vi "Temperature Control.vi"() -> ()   [LabVIEW 2015]
panel:
  out "Warning":bool
  in  "High Limit":dbl
  out "Temperature History":cluster{dbl, "Temp":dbl}(graph)
  in  "Power":bool=TRUE
  # "On"
  # "Off"
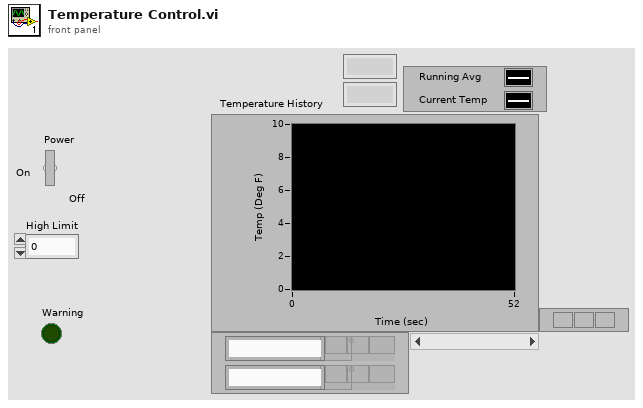
[diagram p1: front panel]
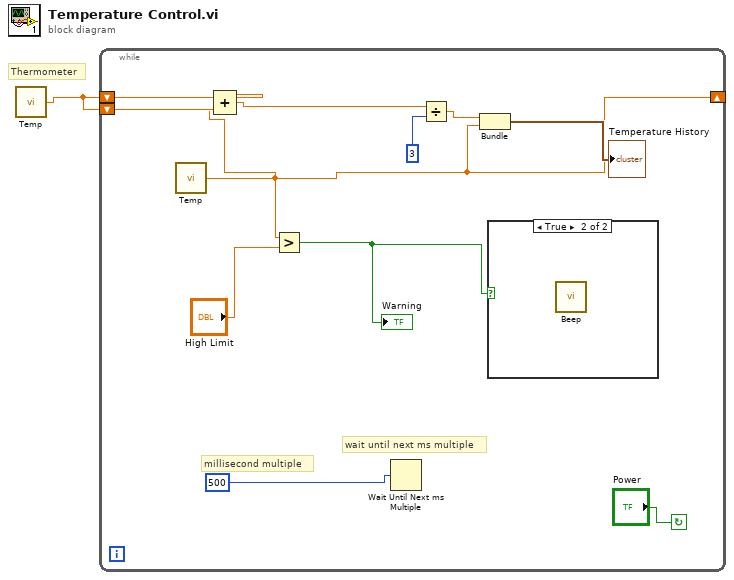
[diagram p0: block diagram]
diagram:
  # "Thermometer"
  n1 = call "Temp.vi"() -> ("Temp"=w1:dbl)  [unwired: 2 in]
  n2 = while {
    shift-right: [w4] -> _
    shift-left: w1 -> [w10]
    shift-left: w1 -> [w9]
    stop <- "Power" continue-if-true
    # "wait until next ms multiple"
    # "millisecond multiple"
    n3 = call "Temp.vi"() -> ("Temp"=w4:dbl)  [unwired: 2 in]
    n4 = Compound Arithmetic op=ADD(w10, w9, w4) -> (w7:dbl)
    n5 = Greater?(x=w4, y="High Limit") -> (0:w2:bool)
    "Warning" <- w2
    n6 = Wait Until Next ms Multiple(millisecond multiple=500) -> ()  [unwired: 1 out]
    n7 = Divide(x=w7, y=3) -> (x/y=w6:dbl)
    n8 = Bundle(w6, "Temp"=w4) -> (→"Temperature History":cluster{dbl, "Temp":dbl})  [unwired: 1 in]
    n9 = case shown="True" w2 {
      frame False {
      }
      frame True {
        n10 = call <vilib>:"Beep.vi"() -> ()  [unwired: 12 in]
      }
    }
  }
